vi "JC_IG4500_configure.vi"(11 "VISA IN (Default COM9)":refnum<visa-resource-name>="COM9") -> (2 "Error":errorcluster, 3 "VISA resource name out":refnum<visa-resource-name>="COM9")   [LabVIEW 2013]
uses:
  <vilib>/Instr/_visa.llb/VISA Configure Serial Port (Instr).vi
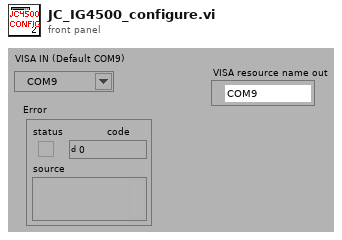
[diagram p1: front panel]
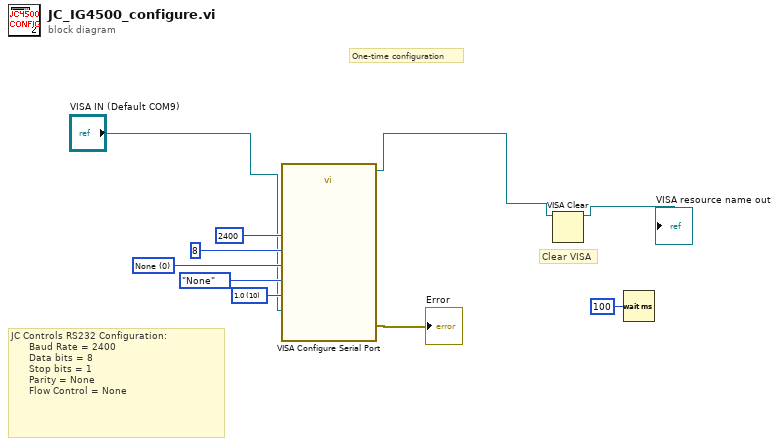
[diagram p0: block diagram]
diagram:
  w8 = u16 0 items=["None", "XON/XOFF", "RTS/CTS", "XON/XOFF & RTS/CTS", "DTR/DSR", "XON/XOFF & DTR/DSR"] ("flow control (0:none)")
  w7 = u16 10 items=["1.0"=10, "1.5"=15, "2.0"=20] ("stop bits (10: 1 bit)")
  # "JC Controls RS232 Configuration:\n      Baud Rate = 2400\n      Data bits = 8\n      Stop bits = 1\n      Parity = None\n      Flow Control = None"
  # "Clear VISA"
  # "One-time configuration"
  n1 = call-poly "VISA Configure Serial Port"("VISA resource name"="VISA IN (Default COM9)", "baud rate (9600)"=u32 2400 ("baud rate"), "data bits (8)"=u16 8 ("data bits"), "parity (0:none)"=enum16{"None", "Odd", "Even", "Mark", "Space"}."None", "stop bits (10: 1 bit)"=w7, "flow control (0:none)"=w8) -> ("VISA resource name out"=w1:refnum<visa-resource-name>, "error out"=→"Error":errorcluster)  [unwired: 8 in]
  n2 = VISA Clear(VISA resource name=w1) -> (VISA resource name out=→"VISA resource name out":refnum<visa-resource-name>)  [unwired: 1 in, 1 out]
  n3 = Wait (ms)(milliseconds to wait=u32 100) -> ()  [unwired: 1 out]
